vi "MH_SetStopOverflow.vi"(8 "error in (no error)":errorcluster, 9 "stopcount":u32=65535, 10 "StopOnOverflow":bool, 11 "devidx":i32) -> (0 "error out":errorcluster, 3 "return type":i32)   [LabVIEW 2019]
uses:
  <userlib>/MultiHarp150/MH_DllPath_global.vi
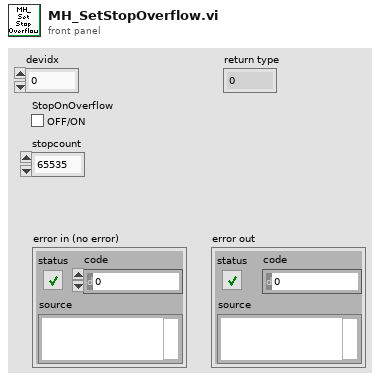
[diagram p1: front panel]
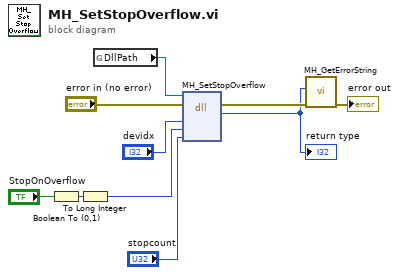
[diagram p0: block diagram]
diagram:
  n1 = Boolean To (0,1)(Boolean="StopOnOverflow") -> (0, 1=w3:i16)
  n2 = To Long Integer(number=w3) -> (32bit integer=w1:i32)
  n3 = global read "MH_DllPath_global.vi" "DllPath"() -> (w9:path)
  n4 = dll-call lib="MHLib64.dll" fn="MH_SetStopOverflow"(path in=w9, error in="error in (no error)", "devidx"="devidx", "StopOnOfl"=w1, "stopcount"="stopcount") -> (error out=w7:errorcluster, "return type"=w6:i32)  [unwired: 4 in, 1 out]
  "return type" <- w6
  n5 = call <userlib>:"MH_GetErrorString.vi"("error in (no error)"=w7, "code"=w6) -> ("error out"=→"error out":errorcluster)  [unwired: 7 in, 2 out]
